vi "Write Section - Timestamp.vi"(5 "format string":string="%<%m/%d/%Y>T", 6 "Create file if not found? (T)":bool=TRUE, 7 "Value":timestamp, 8 "error in (no error)":errorcluster, 9 "key":string, 10 "section":string, 11 "Path":path) -> (0 "error out":errorcluster)   [LabVIEW 2019, in "TSC File IO.lvlib"]
doc: "This VI will write a section/key configuration file of the type:\n<b>Timestamp</b>\n\nInputs:\n-Path [path] - a path to the file\n-section [string] - the section string in the configuration file\n-key [string] - the key to be read in the configuration file\n-value [Timestamp] - the output data written\n-error in\n\nOutputs:\n-error out\n\n<b>Code Developed By:</b>\nDaniel Coons\nTechnology Service Corporation\n1983 S Liberty Drive\nBloomington, IN 47403\nwww.tsc.com\\atcs"
uses:
  TSC File IO.lvlib
  <vilib>/Utility/config.llb/Write Key (String).vi
  <vilib>/Utility/config.llb/NI_LVConfig.lvlib
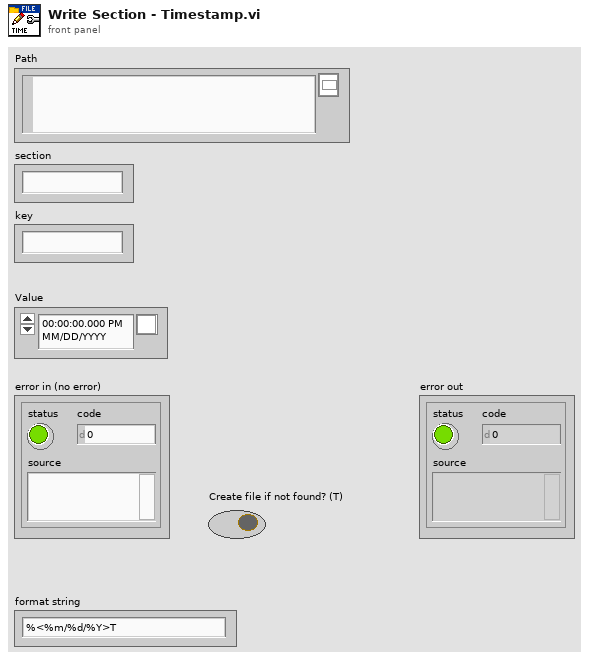
[diagram p1: front panel]
types:
  T1 = typedef "NI_LVConfig.lvlib/Config Data RefNum.ctl" = refnum<k1>
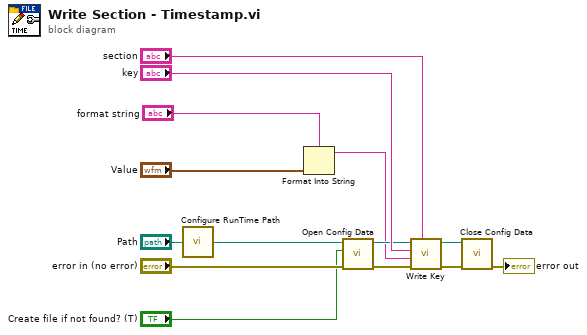
[diagram p0: block diagram]
diagram:
  n1 = call "Configure RunTime Path.vi"("Input Path"="Path") -> ("Updated Path"=w6:path)
  n2 = Format Into String(format string="format string", "Value") -> (resulting string=w2:string)  [unwired: 2 in, 1 out]
  n3 = call <vilib>:"Open Config Data.vi"("error in (no error)"="error in (no error)", "create file if necessary (T)"="Create file if not found? (T)", "configuration file path"=w6) -> ("error out"=w7:errorcluster, "refnum"=w8:T1)  [unwired: 6 in, 1 out]
  n4 = call-poly <vilib>:"Write Key.vi"("section"="section", "error in (no error)"=w7, "value"=w2, "key"="key", "refnum"=w8) -> ("error out"=w9:errorcluster, "refnum out"=w10:T1)  [unwired: 4 in, 1 out]
  n5 = call <vilib>:"Close Config Data.vi"("error in (no error)"=w9, "refnum"=w10) -> ("error out"=→"error out":errorcluster)  [unwired: 8 in, 1 out]
